vi "M08 Energy Storage.vi"(11 "NXT/EV3":T1) -> (3 "EV3 out":T1)   [LabVIEW 2016]
uses:
  <vilib>/NXT/Subs/LVHSConnector.ctl
  <vilib>/NXT/LegoClasses/BrickReference/BrickReference.lvclass
  <vilib>/NXT/Dual Mode Library/Waits/Wait_Num.vi
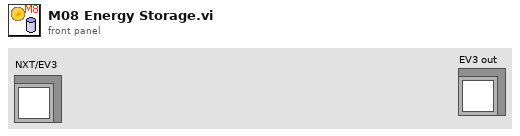
[diagram p1: front panel]
types:
  T1 = typedef "LVHSConnector.ctl" = refnum<class "BrickReference.lvclass">
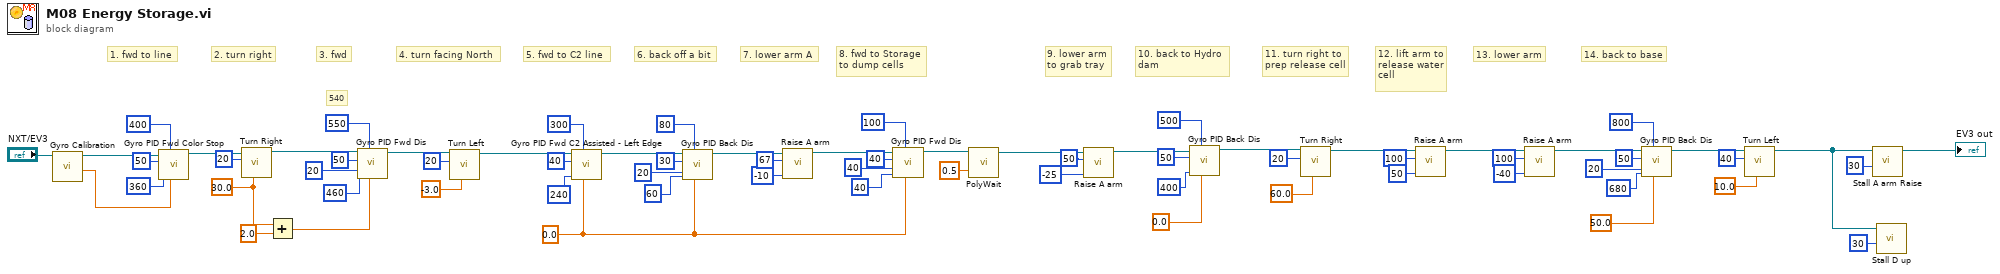
[diagram p0: block diagram]
diagram:
  w34 = sgl 0.0 ("Target angle")
  w37 = sgl 30.0 ("Turning angle")
  # "14. back to base"
  # "13. lower arm"
  # "12. lift arm to\nrelease water\ncell"
  # "11. turn right to\nprep release cell"
  # "10. back to Hydro\ndam"
  # "9. lower arm\nto grab tray"
  # "540"
  # "8. fwd to Storage\nto dump cells"
  # "7. lower arm A"
  # "6. back off a bit"
  # "5. fwd to C2 line"
  # "4. turn facing North"
  # "3. fwd"
  # "2. turn right"
  # "1. fwd to line"
  n1 = call "Gyro Calibration.vi"("NXT/EV3"="NXT/EV3") -> ("Degrees"=w66:sgl, "NXT/EV3"=w27:T1)  [unwired: 6 in, 1 out]
  n2 = call "Gyro PID Fwd Color Stop.vi"("Target angle"=w66, "Threshold to Color"=400, "Threshold to slow"=360, "Max. speed"=50, "EV3 in"=w27) -> ("EV3 out"=w65:T1)  [unwired: 6 in]
  n3 = call "Turn Right.vi"("Turning angle"=w37, "Motor B (right)"=i8 20, "EV3 in"=w65) -> ("EV3 out"=w63:T1)  [unwired: 8 in]
  n4 = Add(x=w37, y=sgl 2.0) -> (x+y=w35:sgl)
  n5 = call "Gyro PID Fwd Dis.vi"("Target angle"=w35, "Threshold to stop"=550, "Threshold to slow"=460, "Min. speed"=20, "Max. speed"=50, "EV3 in"=w63) -> ("EV3 out"=w58:T1)  [unwired: 5 in]
  n6 = call "Turn Left.vi"("Turning angle"=sgl -3.0, "Motor B (right)"=i8 20, "EV3 in"=w58) -> ("EV3 out"=w55:T1)  [unwired: 8 in]
  n7 = call "Gyro PID Fwd C2 Assisted - Left Edge.vi"("Target angle"=w34, "Threshold to Color"=300, "Threshold to slow"=240, "Max. speed"=40, "EV3 in"=w55) -> ("EV3 out"=w51:T1)  [unwired: 6 in]
  n8 = call "Gyro PID Back Dis.vi"("Target angle"=w34, "Threshold to stop"=80, "Threshold to slow"=60, "Min. speed"=20, "Max. speed"=30, "EV3 in"=w51) -> ("EV3 out"=w46:T1)  [unwired: 5 in]
  n9 = call "Raise A arm.vi"("Power"=i8 -10, "Rotation"=67, "EV3 in"=w46) -> ("EV3 out"=w25:T1)  [unwired: 8 in]
  n10 = call "Gyro PID Fwd Dis.vi"("Target angle"=w34, "Threshold to stop"=100, "Threshold to slow"=40, "Min. speed"=40, "Max. speed"=40, "EV3 in"=w25) -> ("EV3 out"=w39:T1)  [unwired: 5 in]
  n11 = call-poly <vilib>:"PolyWait.vi"("Time (1 sec)"=sgl 0.5, "NXT/EV3"=w39) -> ("NXT/EV3"=w17:T1)  [unwired: 2 in]
  n12 = call "Raise A arm.vi"("Power"=i8 -25, "Rotation"=50, "EV3 in"=w17) -> ("EV3 out"=w30:T1)  [unwired: 8 in]
  n13 = call "Gyro PID Back Dis.vi"("Target angle"=sgl 0.0, "Threshold to stop"=500, "Threshold to slow"=400, "Max. speed"=50, "EV3 in"=w30) -> ("EV3 out"=w23:T1)  [unwired: 6 in]
  n14 = call "Turn Right.vi"("Turning angle"=sgl 60.0, "Motor B (right)"=i8 20, "EV3 in"=w23) -> ("EV3 out"=w18:T1)  [unwired: 8 in]
  n15 = call "Raise A arm.vi"("Power"=i8 50, "Rotation"=100, "EV3 in"=w18) -> ("EV3 out"=w10:T1)  [unwired: 8 in]
  n16 = call "Raise A arm.vi"("Power"=i8 -40, "Rotation"=100, "EV3 in"=w10) -> ("EV3 out"=w9:T1)  [unwired: 8 in]
  n17 = call "Gyro PID Back Dis.vi"("Target angle"=sgl 50.0, "Threshold to stop"=800, "Threshold to slow"=680, "Min. speed"=20, "Max. speed"=50, "EV3 in"=w9) -> ("EV3 out"=w5:T1)  [unwired: 5 in]
  n18 = call "Turn Left.vi"("Turning angle"=sgl 10.0, "Motor B (right)"=i8 40, "EV3 in"=w5) -> ("EV3 out"=w3:T1)  [unwired: 8 in]
  n19 = call "Stall A arm Raise.vi"("Power"=i8 30, "NXT/EV3"=w3) -> ("NXT/EV3"=→"EV3 out":T1)  [unwired: 9 in]
  n20 = call "Stall D up.vi"("Power"=i8 30, "NXT/EV3"=w3) -> ()  [unwired: 9 in, 1 out]
